vi "TestiLabviewLIVELowLevel.vi"() -> ()   [LabVIEW 2018]
uses:
  <vilib>/vision/Image Controls.llb/IMAQ Image.ctl
  <vilib>/vision/NI_Vision_Development_Module.lvlib
  <vilib>/vision/driver/NI_Vision_Acquisition_Software.lvlib
panel:
  out "Image 5":T1(plugin-control)
  out "Y 4":dbl[](array[numeric])
  out "X 4":dbl[](array[numeric])
  out "Antal isbjerg 4":i32
  out "status":bool
  out "x .or. y?":bool
  out "Numeric":i32
  out "Image 4":T1(plugin-control)
  out "Antal isbjerg 3":i32
  out "X 3":dbl[](array[numeric])
  out "Y 3":dbl[](array[numeric])
  in  "Range":cluster{"Lower value":sgl, "Upper value":sgl}={"Lower value"=245.0, "Upper value"=250.0}
  out "Y 2":dbl[](array[numeric])
  out "X 2":dbl[](array[numeric])
  out "Antal isbjerg 2":i32
  out "Antal isbjerg":i32
  out "X":dbl[](array[numeric])
  out "Y":dbl[](array[numeric])
  in  "Stop (F)":bool
  # "Tager isbjerge i rækkefølgen: y: 0 -> max"
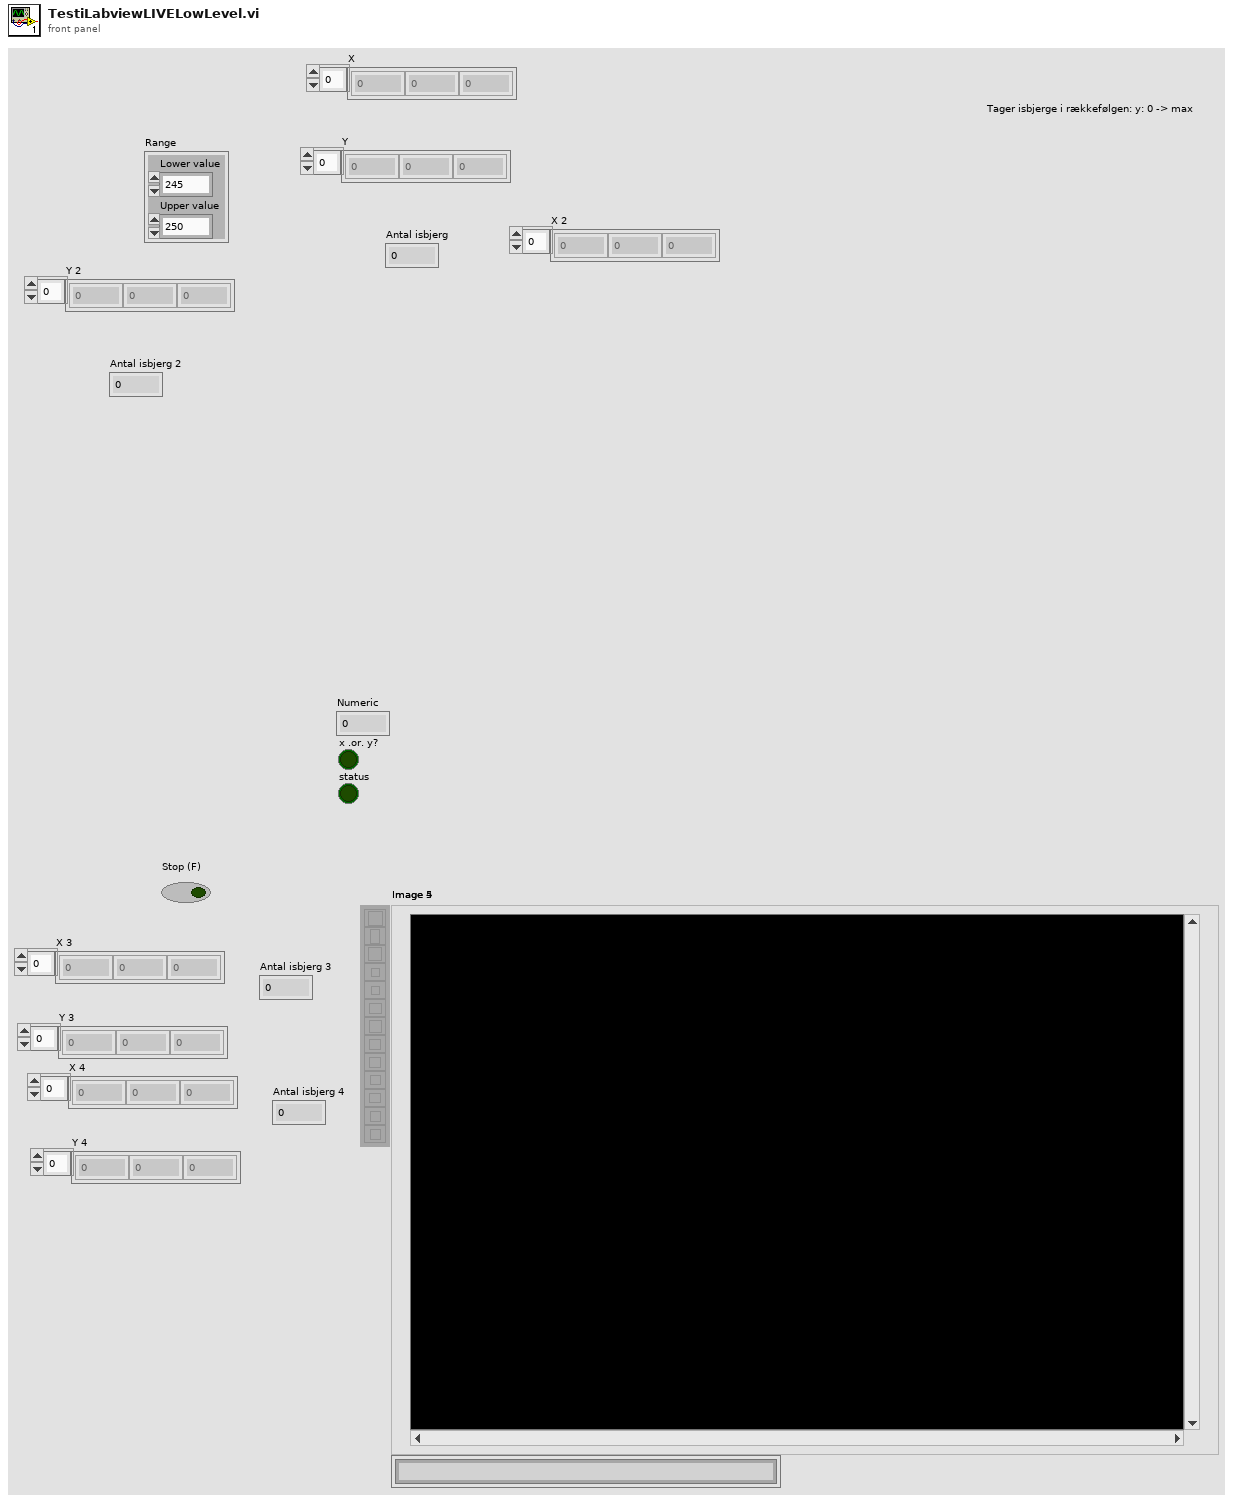
[diagram p1: front panel]
types:
  T1 = typedef "IMAQ Image.ctl" = refnum<image>
  T2 = enum32{"AutoM", "Close", "Dilate", "Erode", "Gradient", "Gradient out", "Gradient in", "Hit miss", "Open", "PClose", "POpen", "Thick", "Thin"}
  T3 = typedef "Image Type" = u32
  T4 = typedef "IMAQdx.ctl" = refnum<k21>
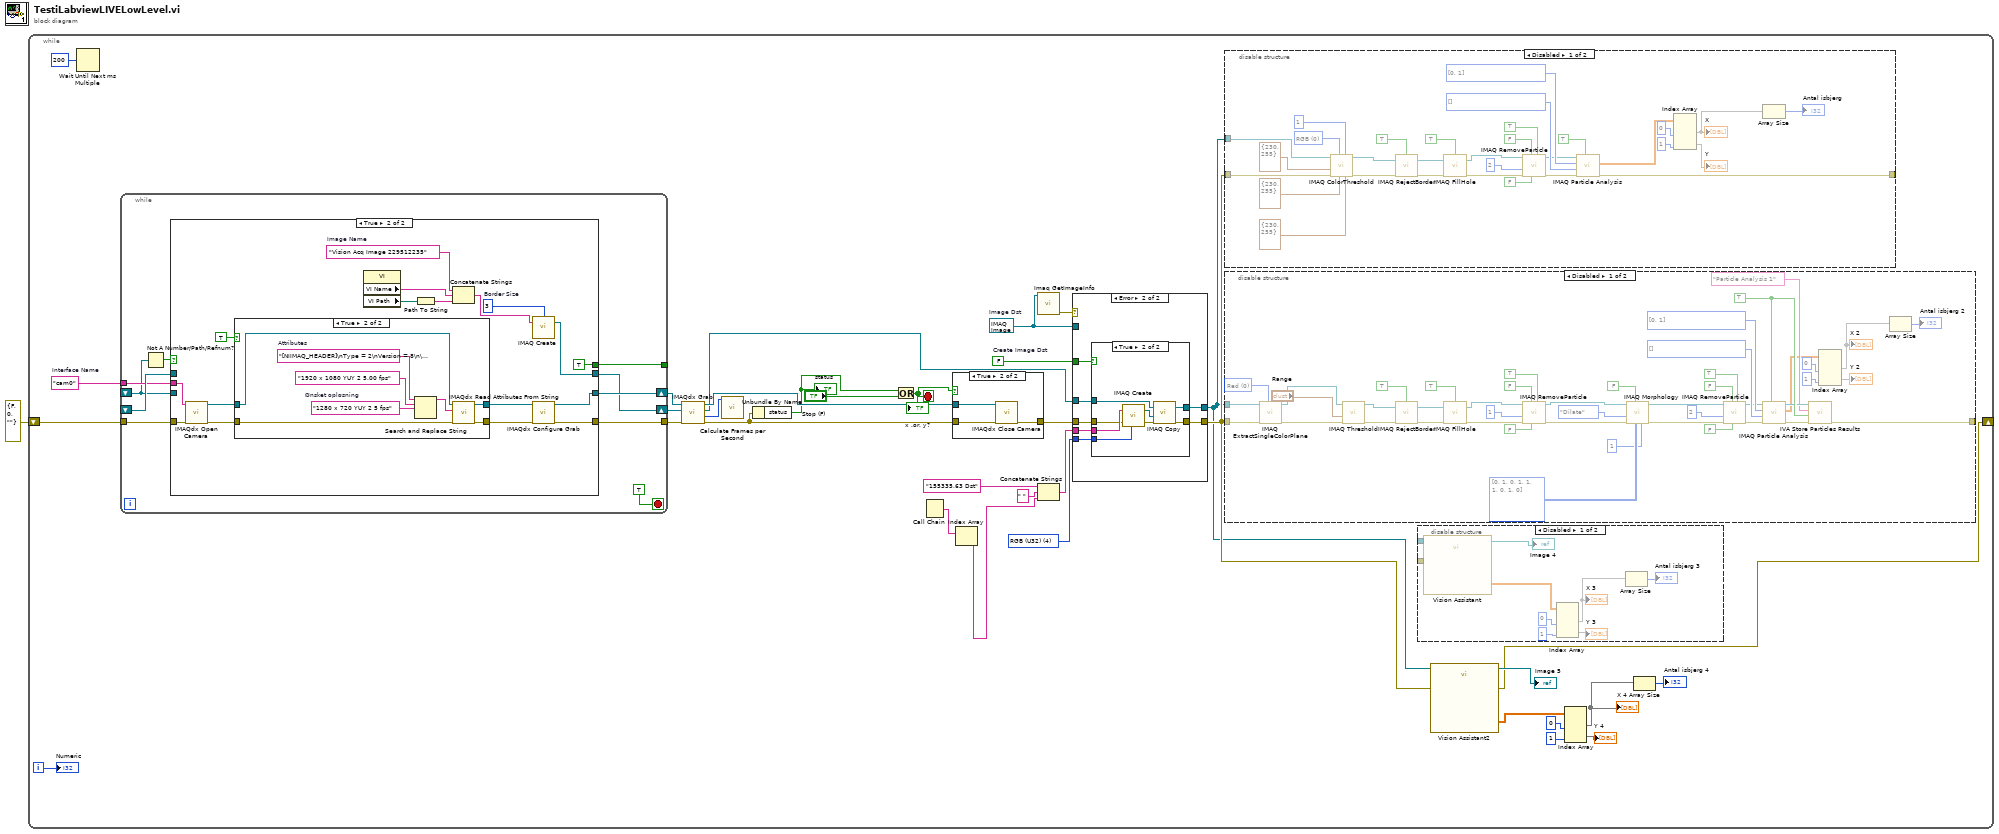
[diagram p0: block diagram]
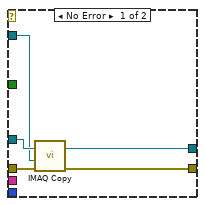
[diagram p8: hidden frame]
diagram:
  n1 = while {
    shift-right: [w4] -> _
    shift-left: errorcluster {"status"=FALSE, "code"=0, "source"=""} ("error in") -> [w17]
    i -> [w13]
    stop <- w19 stop-if-true
    w25 = "cam0"  # Interface Name
    w35 = T1 refnum  # Image Dst
    w27 = T3 4 items=["Grayscale (U8)", "Grayscale (I16)", "Grayscale (SGL)", "Complex (CSG)", "RGB (U32)", "HSL (U32)", "RGB (U64)", "Grayscale (U16)"] ("Image Dst Type")
    w33 = FALSE  # Create Image Dst
    n2 = Wait Until Next ms Multiple(millisecond multiple=u32 200) -> ()  [unwired: 1 out]
    n3 = while "While Loop_template0" {
      shift-right: [w136] -> w15
      shift-left: _ -> [w129]
      tunnel: [w135] -> w26
      tunnel: w17 -> [w134]
      shift-right: [w132] -> w16
      shift-left: _ -> [w131]
      tunnel: w25 -> [w130]
      tunnel: [w127] -> _
      stop <- TRUE ("_template0") stop-if-true
      n4 = Not A Number/Path/Refnum?(number/path/refnum=w129) -> (NaN/Path/Refnum?=w128:bool)
      n5 = case "Case Structure_template0" shown="True" w128 {
        tunnel: [w139 w155] -> w136
        tunnel: w129 -> [w139 _]
        tunnel: [w138 w154] -> w135
        tunnel: w134 -> [w138 w156]
        tunnel: [w137 w153] -> w132
        tunnel: w131 -> [w137 _]
        tunnel: w130 -> [_ w143]
        tunnel: [_ TRUE] -> w127
        frame False {
        }
        frame True {
          w140 = 3  # Border Size
          w148 = "Vision Acq Image 229512235"  # Image Name
          n6 = call <vilib>:"IMAQdx Open Camera.vi"("error in"=w156, "Session In"=w143) -> ("error out"=w146:errorcluster, "Session Out"=w147:T4)  [unwired: 1 in, 7 out]
          n7 = case shown="True" TRUE ("Init Attributes") {
            tunnel: w147 -> [w158 w166]
            tunnel: w146 -> [w157 w165]
            tunnel: [w158 w164] -> w145
            tunnel: [w157 w163] -> w144
            frame False {
            }
            frame True {
              w159 = "1280 x 720 YUY 2 5 fps"  # Ønsket opløsning
              w162 = "[NIIMAQ_HEADER]\nType = 2\nVersion = 8\n\n[CAMERA_DATA]\nAcquisitionAttributes::Bayer::Algorithm = \"Bilinear\"\nAcquisitionAttributes::Bayer::GainB = \"1\"\nAcquisitionAttributes::Bayer::GainG = \"1\"\nAcquisitionAttributes::Bayer::GainR = \"1\"\nAcquisitionAttributes::Bayer::Pattern = \"Use hardware value\"\nAcquisitionAttributes::BitsPerPixel = \"Use hardware value\"\nAcquisitionAttributes::HardwareMaximumQueuedBufferCount = \"1000\"\nAcquisitionAttributes::HardwareRequeueBufferListThreshold = \"50\"\nAcquisitionAttributes::IgnoreFirstFrame = \"false\"\nAcquisitionAttributes::ImageDecoderCopyMode = \"Auto\"\nAcquisitionAttributes::OutputImageType = \"Auto\"\nAcquisitionAttributes::OverwriteMode = \"Get Newest\"\nAcquisitionAttributes::PixelSignedness = \"Use hardware value\"\nAcquisitionAttributes::ReceiveTimestampMode = \"None\"\nAcquisitionAttributes::ShiftPixelBits = \"false\"\nAcquisitionAttributes::SwapPixelBytes = \"false\"\nAcquisitionAttributes::Timeout = \"5000\"\nAcquisitionAttributes::VideoMode = \"1920 x 1080 YUY 2 5.00 fps\"\nCameraAttributes::BacklightCompensation::Mode = \"Manual\"\nCameraAttributes::BacklightCompensation::Value = \"0\"\nCameraAttributes::Brightness::Mode = \"Manual\"\nCameraAttributes::Brightness::Value = \"168\"\nCameraAttributes::Contrast::Mode = \"Manual\"\nCameraAttributes::Contrast::Value = \"5\"\nCameraAttributes::Exposure::Mode = \"AutoAperaturePriority\"\nCameraAttributes::Focus::Mode = \"Auto\"\nCameraAttributes::Pan::Mode = \"Manual\"\nCameraAttributes::Pan::Value = \"0\"\nCameraAttributes::PowerLineFrequency::Mode = \"60Hz\"\nCameraAttributes::Saturation::Mode = \"Manual\"\nCameraAttributes::Saturation::Value = \"103\"\nCameraAttributes::Sharpness::Mode = \"Manual\"\nCameraAttributes::Sharpness::Value = \"25\"\nCameraAttributes::Tilt::Mode = \"Manual\"\nCameraAttributes::Tilt::Value = \"0\"\nCameraAttributes::WhiteBalance::Mode = \"Auto\"\nCameraAttributes::Zoom::Mode = \"Manual\"\nCameraAttributes::Zoom::Value = \"0\"\n"  # Attributes
              n8 = Search and Replace String(input string=w162, search string="1920 x 1080 YUY 2 5.00 fps", replace string=w159) -> (result string=w160:string)  [unwired: 5 in, 3 out]
              n9 = call <vilib>:"IMAQdx Read Attributes From String.vi"("error in"=w165, "Attributes String In"=w160, "Session In"=w166) -> ("error out"=w163:errorcluster, "Session Out"=w164:T4)  [unwired: 7 out]
            }
          }
          n10 = property class="VI"() -> ("VI Name"=w151:string, "VI Path"=w152:path)  [unwired: 2 in, 2 out]
          n11 = Path To String(path=w152) -> (string=w150:string)
          n12 = Concatenate Strings(w148, w151, w150) -> (w149:string)
          n13 = call "IMAQ Create"("Border Size"=w140, "Image Name"=w149) -> ("New Image"=w153:T1)  [unwired: 2 in, 2 out]
          n14 = call <vilib>:"IMAQdx Configure Grab.vi"("error in"=w144, "Session In"=w145) -> ("error out"=w154:errorcluster, "Session Out"=w155:T4)  [unwired: 8 out]
        }
      }
    }
    n15 = call <vilib>:"IMAQdx Grab.vi"("error in"=w26, "Image In"=w16, "Session In"=w15) -> ("error out"=w24:errorcluster, "Buffer Number Out"=w23:u32, "Image Out"=w2:T1, "Session Out"=w22:T4)  [unwired: 1 in, 4 out]
    n16 = call <vilib>:"Calculate Frames per Second.vi"("Buffer Number"=w23) -> ()  [unwired: 2 in, 9 out]
    n17 = Unbundle By Name(w24) -> ("status"=w14:bool)
    "status" <- w14
    n18 = Or(x=w14, y="Stop (F)") -> (x .or. y?=w19:bool)
    "x .or. y?" <- w19
    n19 = Call Chain() -> (call chain=w32:string[])
    n20 = case "Case Structure_template1" shown="True" w19 {
      tunnel: [w123 w125] -> w20
      tunnel: w24 -> [w123 w126]
      tunnel: w22 -> [_ w124]
      frame False {
      }
      frame True {
        n21 = call <vilib>:"IMAQdx Close Camera.vi"("error in"=w126, "Session In"=w124) -> ("error out"=w125:errorcluster)  [unwired: 9 out]
      }
    }
    n22 = Index Array(array=w32) -> (element=w30:string)  [unwired: 1 in]
    n23 = call "Imaq GetImageInfo"("Image"=w35) -> ("error out"=w34:errorcluster)  [unwired: 1 in, 9 out]
    n24 = Concatenate Strings("155335,63 Dst" ("Image Dst Name"), " ", w30) -> (w28:string)
    n25 = case shown="Error" w34 {
      tunnel: [w171 w175] -> w3
      tunnel: [w170 w174] -> w5
      tunnel: w2 -> [w169 w176]
      tunnel: w20 -> [w168 w172]
      tunnel: w35 -> [w167 _]
      tunnel: w28 -> [_ w178]
      tunnel: w27 -> [_ w177]
      tunnel: w33 -> [_ w173]
      frame No Error {
        n26 = call "IMAQ Copy"("error in (no error)"=w168, "Image Dst"=w167, "Image Src"=w169) -> ("error out"=w170:errorcluster, "Image Dst Out"=w171:T1)  [unwired: 3 out]
      }
      frame Error {
        n27 = case shown="True" w173 {
          tunnel: w178 -> [_ w188]
          tunnel: w177 -> [_ w187]
          tunnel: w176 -> [w180 w185]
          tunnel: [w180 w184] -> w175
          tunnel: [w179 w183] -> w174
          tunnel: w172 -> [w179 w181]
          frame False {
          }
          frame True {
            n28 = call "IMAQ Create"("Image Name"=w188, "Image Type"=w187, "error in (no error)"=w181) -> ("New Image"=w186:T1, "error out"=w182:errorcluster)  [unwired: 1 in, 1 out]
            n29 = call "IMAQ Copy"("error in (no error)"=w182, "Image Dst"=w186, "Image Src"=w185) -> ("error out"=w183:errorcluster, "Image Dst Out"=w184:T1)  [unwired: 3 out]
          }
        }
      }
    }
    n30 = disable-structure shown="Disabled" {
      disable-tunnel: w5 -> [w56 _]
      disable-tunnel: [w49 _] -> _
      disable-tunnel: w3 -> [w46 _]
      frame Disabled {
        w61 = i32[] [] items=["Center of Mass X", "Center of Mass Y", "First Pixel X", "First Pixel Y", "Bounding Rect Left", "Bounding Rect Top", "Bounding Rect Right", "Bounding Rect Bottom", "Max Feret Diameter Start X", "Max Feret Diameter Start Y", "Max Feret Diameter End X", "Max Feret Diameter End Y", "Max Horiz. Segment Length Left", "Max Horiz. Segment Length Right", "Max Horiz. Segment Length Row", "-", "Bounding Rect Width", "Bounding Rect Height", "Bounding Rect Diagonal", "Perimeter", "Convex Hull Perimeter", "Holes' Perimeter", "Max Feret Diameter", "Equivalent Ellipse Major Axis", "Equivalent Ellipse Minor Axis", "Equivalent Ellipse Minor Axis (Feret)", "Equivalent Rect Long Side", "Equivalent Rect Short Side", "Equivalent Rect Diagonal", "Equivalent Rect Short Side (Feret)", "Average Horiz. Segment Length", "Average Vert. Segment Length", "Hydraulic Radius", "Waddel Disk Diameter", "-", "Area", "Holes' Area", "Particle & Holes' Area", "Convex Hull Area", "Image Area", "-", "Number of Holes", "Number of Horiz. Segments", "Number of Vert. Segments", "-", "Orientation", "Max Feret Diameter Orientation", "-", "% Area/Image Area", "% Area/(Particle & Holes' Area)", "Ratio of Equivalent Ellipse Axes", "Ratio of Equivalent Rect Sides", "-", "Elongation Factor", "Compactness Factor", "Heywood Circularity Factor", "Type Factor", "-", "Sum X", "Sum Y", "Sum XX", "Sum XY", "Sum YY", "Sum XXX", "Sum XXY", "Sum XYY", "Sum YYY", "-", "Moment of Inertia XX", "Moment of Inertia XY", "Moment of Inertia YY", "Moment of Inertia XXX", "Moment of Inertia XXY", "Moment of Inertia XYY", "Moment of Inertia YYY", "Norm. Moment of Inertia XX", "Norm. Moment of Inertia XY", "Norm. Moment of Inertia YY", "Norm. Moment of Inertia XXX", "Norm. Moment of Inertia XXY", "Norm. Moment of Inertia XYY", "Norm. Moment of Inertia YYY", "Hu Moment 1", "Hu Moment 2", "Hu Moment 3", "Hu Moment 4", "Hu Moment 5", "Hu Moment 6", "Hu Moment 7"] ("Real-World Measurements")
        w62 = i32[] [0, 1] items=["Center of Mass X", "Center of Mass Y", "First Pixel X", "First Pixel Y", "Bounding Rect Left", "Bounding Rect Top", "Bounding Rect Right", "Bounding Rect Bottom", "Max Feret Diameter Start X", "Max Feret Diameter Start Y", "Max Feret Diameter End X", "Max Feret Diameter End Y", "Max Horiz. Segment Length Left", "Max Horiz. Segment Length Right", "Max Horiz. Segment Length Row", "-", "Bounding Rect Width", "Bounding Rect Height", "Bounding Rect Diagonal", "Perimeter", "Convex Hull Perimeter", "Holes' Perimeter", "Max Feret Diameter", "Equivalent Ellipse Major Axis", "Equivalent Ellipse Minor Axis", "Equivalent Ellipse Minor Axis (Feret)", "Equivalent Rect Long Side", "Equivalent Rect Short Side", "Equivalent Rect Diagonal", "Equivalent Rect Short Side (Feret)", "Average Horiz. Segment Length", "Average Vert. Segment Length", "Hydraulic Radius", "Waddel Disk Diameter", "-", "Area", "Holes' Area", "Particle & Holes' Area", "Convex Hull Area", "Image Area", "-", "Number of Holes", "Number of Horiz. Segments", "Number of Vert. Segments", "-", "Orientation", "Max Feret Diameter Orientation", "-", "% Area/Image Area", "% Area/(Particle & Holes' Area)", "Ratio of Equivalent Ellipse Axes", "Ratio of Equivalent Rect Sides", "-", "Elongation Factor", "Compactness Factor", "Heywood Circularity Factor", "Type Factor", "-", "Sum X", "Sum Y", "Sum XX", "Sum XY", "Sum YY", "Sum XXX", "Sum XXY", "Sum XYY", "Sum YYY", "-", "Moment of Inertia XX", "Moment of Inertia XY", "Moment of Inertia YY", "Moment of Inertia XXX", "Moment of Inertia XXY", "Moment of Inertia XYY", "Moment of Inertia YYY", "Norm. Moment of Inertia XX", "Norm. Moment of Inertia XY", "Norm. Moment of Inertia YY", "Norm. Moment of Inertia XXX", "Norm. Moment of Inertia XXY", "Norm. Moment of Inertia XYY", "Norm. Moment of Inertia YYY", "Hu Moment 1", "Hu Moment 2", "Hu Moment 3", "Hu Moment 4", "Hu Moment 5", "Hu Moment 6", "Hu Moment 7"] ("Pixel Measurements")
        w60 = TRUE ("Connectivity 4/8 (8)")
        w91 = 0 items=["Red", "Green", "Blue", "Hue", "Saturation", "Luminance", "Value", "Intensity"] ("Color Plane")
        n31 = call "IMAQ ExtractSingleColorPlane"("Color Plane"=w91, "error in (no error)"=w56, "Image Src"=w46) -> ("error out"=w90:errorcluster, "Image Dst Out"=w88:T1)  [unwired: 1 in, 6 out]
        n32 = call "IMAQ Threshold"("error in (no error)"=w90, "Range"="Range", "Image Src"=w88) -> ("error out"=w87:errorcluster, "Image Dst Out"=w85:T1)  [unwired: 3 in, 4 out]
        n33 = call "IMAQ RejectBorder"("error in (no error)"=w87, "Image Src"=w85, "Connectivity 4/8 (8)"=TRUE) -> ("error out"=w84:errorcluster, "Image Dst Out"=w82:T1)  [unwired: 1 in, 2 out]
        n34 = call "IMAQ FillHole"("error in (no error)"=w84, "Image Src"=w82, "Connectivity 4/8 (8)"=TRUE) -> ("error out"=w81:errorcluster, "Image Dst Out"=w76:T1)  [unwired: 1 in, 2 out]
        n35 = call "IMAQ RemoveParticle"("Connectivity 4/8 (8)"=TRUE, "Low Pass/High Pass (Low)"=FALSE, "Square/Hexa (Square)"=FALSE, "error in (no error)"=w81, "Number of Erosion"=1, "Image Src"=w76) -> ("error out"=w75:errorcluster, "Image Dst Out"=w70:T1)  [unwired: 1 in, 3 out]
        n36 = call "IMAQ Morphology"("Number of iterations (1)"=1, "Structuring Element"=i32[][] [[0, 1, 0], [1, 1, 1], [0, 1, 0]], "Square/Hexa (Square)"=FALSE, "error in (no error)"=w75, "Operation"=T2."Dilate", "Image Src"=w70) -> ("error out"=w69:errorcluster, "Image Dst Out"=w64:T1)  [unwired: 1 in, 3 out]
        n37 = call "IMAQ RemoveParticle"("Connectivity 4/8 (8)"=TRUE, "Low Pass/High Pass (Low)"=FALSE, "Square/Hexa (Square)"=FALSE, "error in (no error)"=w69, "Number of Erosion"=2, "Image Src"=w64) -> ("error out"=w63:errorcluster, "Image Dst Out"=w47:T1)  [unwired: 1 in, 3 out]
        n38 = call "IMAQ Particle Analysis"("Connectivity 4/8 (8)"=w60, "error in (no error)"=w63, "Real-World Measurements"=w61, "Pixel Measurements"=w62, "Image"=w47) -> ("error out"=w57:errorcluster, "Particle Measurements (Pixels)"=w50:dbl[][], "Image Out (duplicate)"=w59:T1)  [unwired: 4 out]
        n39 = call <vilib>:"IVA Store Particles Results.vi"("error in (no error)"=w57, "Connectivity 4/8 (8)"=w60, "Step Name"="Particle Analysis 1", "Image in"=w59) -> ("error out"=w49:errorcluster, "Image dup"=w48:T1)  [unwired: 6 out]
        n40 = Index Array(array=w50, index (col) #1=0 ("index (col)"), index (col) #2=1 ("index (col)")) -> (element #1=w53:dbl[], element #2=→"Y 2":dbl[])  [unwired: 2 in]
        "X 2" <- w53
        n41 = Array Size(array=w53) -> (size(s)=→"Antal isbjerg 2":i32)
      }
      frame Enabled {
      }
    }
    n42 = disable-structure shown="Disabled" {
      disable-tunnel: [w94 _] -> _
      disable-tunnel: w3 -> [w93 _]
      disable-tunnel: w5 -> [w92 _]
      frame Disabled {
        w99 = i32[] [] items=["Center of Mass X", "Center of Mass Y", "First Pixel X", "First Pixel Y", "Bounding Rect Left", "Bounding Rect Top", "Bounding Rect Right", "Bounding Rect Bottom", "Max Feret Diameter Start X", "Max Feret Diameter Start Y", "Max Feret Diameter End X", "Max Feret Diameter End Y", "Max Horiz. Segment Length Left", "Max Horiz. Segment Length Right", "Max Horiz. Segment Length Row", "-", "Bounding Rect Width", "Bounding Rect Height", "Bounding Rect Diagonal", "Perimeter", "Convex Hull Perimeter", "Holes' Perimeter", "Max Feret Diameter", "Equivalent Ellipse Major Axis", "Equivalent Ellipse Minor Axis", "Equivalent Ellipse Minor Axis (Feret)", "Equivalent Rect Long Side", "Equivalent Rect Short Side", "Equivalent Rect Diagonal", "Equivalent Rect Short Side (Feret)", "Average Horiz. Segment Length", "Average Vert. Segment Length", "Hydraulic Radius", "Waddel Disk Diameter", "-", "Area", "Holes' Area", "Particle & Holes' Area", "Convex Hull Area", "Image Area", "-", "Number of Holes", "Number of Horiz. Segments", "Number of Vert. Segments", "-", "Orientation", "Max Feret Diameter Orientation", "-", "% Area/Image Area", "% Area/(Particle & Holes' Area)", "Ratio of Equivalent Ellipse Axes", "Ratio of Equivalent Rect Sides", "-", "Elongation Factor", "Compactness Factor", "Heywood Circularity Factor", "Type Factor", "-", "Sum X", "Sum Y", "Sum XX", "Sum XY", "Sum YY", "Sum XXX", "Sum XXY", "Sum XYY", "Sum YYY", "-", "Moment of Inertia XX", "Moment of Inertia XY", "Moment of Inertia YY", "Moment of Inertia XXX", "Moment of Inertia XXY", "Moment of Inertia XYY", "Moment of Inertia YYY", "Norm. Moment of Inertia XX", "Norm. Moment of Inertia XY", "Norm. Moment of Inertia YY", "Norm. Moment of Inertia XXX", "Norm. Moment of Inertia XXY", "Norm. Moment of Inertia XYY", "Norm. Moment of Inertia YYY", "Hu Moment 1", "Hu Moment 2", "Hu Moment 3", "Hu Moment 4", "Hu Moment 5", "Hu Moment 6", "Hu Moment 7"] ("Real-World Measurements")
        w100 = i32[] [0, 1] items=["Center of Mass X", "Center of Mass Y", "First Pixel X", "First Pixel Y", "Bounding Rect Left", "Bounding Rect Top", "Bounding Rect Right", "Bounding Rect Bottom", "Max Feret Diameter Start X", "Max Feret Diameter Start Y", "Max Feret Diameter End X", "Max Feret Diameter End Y", "Max Horiz. Segment Length Left", "Max Horiz. Segment Length Right", "Max Horiz. Segment Length Row", "-", "Bounding Rect Width", "Bounding Rect Height", "Bounding Rect Diagonal", "Perimeter", "Convex Hull Perimeter", "Holes' Perimeter", "Max Feret Diameter", "Equivalent Ellipse Major Axis", "Equivalent Ellipse Minor Axis", "Equivalent Ellipse Minor Axis (Feret)", "Equivalent Rect Long Side", "Equivalent Rect Short Side", "Equivalent Rect Diagonal", "Equivalent Rect Short Side (Feret)", "Average Horiz. Segment Length", "Average Vert. Segment Length", "Hydraulic Radius", "Waddel Disk Diameter", "-", "Area", "Holes' Area", "Particle & Holes' Area", "Convex Hull Area", "Image Area", "-", "Number of Holes", "Number of Horiz. Segments", "Number of Vert. Segments", "-", "Orientation", "Max Feret Diameter Orientation", "-", "% Area/Image Area", "% Area/(Particle & Holes' Area)", "Ratio of Equivalent Ellipse Axes", "Ratio of Equivalent Rect Sides", "-", "Elongation Factor", "Compactness Factor", "Heywood Circularity Factor", "Type Factor", "-", "Sum X", "Sum Y", "Sum XX", "Sum XY", "Sum YY", "Sum XXX", "Sum XXY", "Sum XYY", "Sum YYY", "-", "Moment of Inertia XX", "Moment of Inertia XY", "Moment of Inertia YY", "Moment of Inertia XXX", "Moment of Inertia XXY", "Moment of Inertia XYY", "Moment of Inertia YYY", "Norm. Moment of Inertia XX", "Norm. Moment of Inertia XY", "Norm. Moment of Inertia YY", "Norm. Moment of Inertia XXX", "Norm. Moment of Inertia XXY", "Norm. Moment of Inertia XYY", "Norm. Moment of Inertia YYY", "Hu Moment 1", "Hu Moment 2", "Hu Moment 3", "Hu Moment 4", "Hu Moment 5", "Hu Moment 6", "Hu Moment 7"] ("Pixel Measurements")
        w117 = u16 0 items=["RGB", "HSL", "HSV", "HSI"] ("Color Mode")
        n43 = call "IMAQ ColorThreshold"("Blue or Luma or Val or Inten Range"=cluster{"Lower value":i32, "Upper value":i32} {"Lower value"=230, "Upper value"=255}, "Replace Value"=1, "Green or Sat Range"=cluster{"Lower value":i32, "Upper value":i32} {"Lower value"=230, "Upper value"=255}, "Color Mode"=w117, "error in (no error)"=w92, "Red or Hue Range"=cluster{"Lower value":i32, "Upper value":i32} {"Lower value"=230, "Upper value"=255}, "Image Src"=w93) -> ("error out"=w113:errorcluster, "Image Dst Out"=w111:T1)  [unwired: 1 in, 2 out]
        n44 = call "IMAQ RejectBorder"("error in (no error)"=w113, "Image Src"=w111, "Connectivity 4/8 (8)"=TRUE) -> ("error out"=w110:errorcluster, "Image Dst Out"=w108:T1)  [unwired: 1 in, 2 out]
        n45 = call "IMAQ FillHole"("error in (no error)"=w110, "Image Src"=w108, "Connectivity 4/8 (8)"=TRUE) -> ("error out"=w107:errorcluster, "Image Dst Out"=w102:T1)  [unwired: 1 in, 2 out]
        n46 = call "IMAQ RemoveParticle"("Connectivity 4/8 (8)"=TRUE, "Low Pass/High Pass (Low)"=FALSE, "Square/Hexa (Square)"=FALSE, "error in (no error)"=w107, "Number of Erosion"=2, "Image Src"=w102) -> ("error out"=w101:errorcluster, "Image Dst Out"=w98:T1)  [unwired: 1 in, 3 out]
        n47 = call "IMAQ Particle Analysis"("Connectivity 4/8 (8)"=TRUE, "error in (no error)"=w101, "Real-World Measurements"=w99, "Pixel Measurements"=w100, "Image"=w98) -> ("error out"=w94:errorcluster, "Particle Measurements (Pixels)"=w96:dbl[][])  [unwired: 5 out]
        n48 = Index Array(array=w96, index (col) #1=0 ("index (col)"), index (col) #2=1 ("index (col)")) -> (element #1=w120:dbl[], element #2=→"Y":dbl[])  [unwired: 2 in]
        "X" <- w120
        n49 = Array Size(array=w120) -> (size(s)=→"Antal isbjerg":i32)
      }
      frame Enabled {
      }
    }
    n50 = disable-structure shown="Disabled" {
      disable-tunnel: _ -> [w45 _]
      disable-tunnel: _ -> [w37 _]
      frame Disabled {
        n51 = call "Vision Assistant"("Image In"=w45, "error in"=w37) -> ("Image Out"=→"Image 4":T1, "Particle Measurements (Pixels) (Particle Analysis 1)"=w41:dbl[][], "error out"=w36:errorcluster)  [unwired: 23 in]
        n52 = Index Array(array=w41, index (col) #1=0 ("index (col)"), index (col) #2=1 ("index (col)")) -> (element #1=w43:dbl[], element #2=→"Y 3":dbl[])  [unwired: 2 in]
        "X 3" <- w43
        n53 = Array Size(array=w43) -> (size(s)=→"Antal isbjerg 3":i32)
      }
      frame Enabled {
      }
    }
    n54 = call "Vision Assistant2"("Image In"=w3, "error in"=w5) -> ("Image Out"=→"Image 5":T1, "Particle Measurements (Pixels) (Particle Analysis 1)"=w7:dbl[][], "error out"=w4:errorcluster)  [unwired: 23 in]
    n55 = Index Array(array=w7, index (col) #1=0 ("index (col)"), index (col) #2=1 ("index (col)")) -> (element #1=w9:dbl[], element #2=→"Y 4":dbl[])  [unwired: 2 in]
    "X 4" <- w9
    n56 = Array Size(array=w9) -> (size(s)=→"Antal isbjerg 4":i32)
    "Numeric" <- w13
  }
